vi "Front Panel Control Example.vi"() -> ()   [LabVIEW 2020]
uses:
  Controls/FP Control Functions.ctl
panel:
  in  "stop":bool
  # "While the VI is running, open the block diagram (Ctrl-E) and wait."
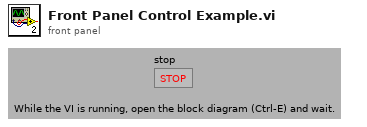
[diagram p1: front panel]
types:
  T1 = typedef "FP Control Functions.ctl" = enum16{"Open", "Close", "Bring To Front", "Center"}
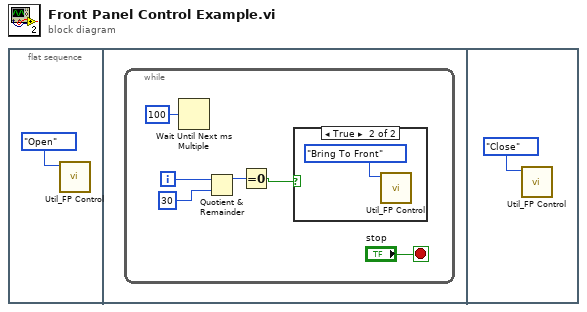
[diagram p0: block diagram]
diagram:
  n1 = flat-sequence {
    frame #0 {
      n2 = call "Util_FP Control.vi"("Function"=FP_Control_Functions."Open") -> ()  [unwired: 1 in, 10 out]
    }
    frame #1 {
      n3 = while {
        i -> [w5]
        stop <- "stop" stop-if-true
        n4 = Wait Until Next ms Multiple(millisecond multiple=u32 100) -> ()  [unwired: 1 out]
        n5 = Quotient & Remainder(x=w5, y=30) -> (x-y*floor(x/y)=w3:i32)  [unwired: 1 out]
        n6 = Equal To 0?(x=w3) -> (x = 0?=w2:bool)
        n7 = case shown="True" w2 {
          frame False {
          }
          frame True {
            n8 = call "Util_FP Control.vi"("Function"=FP_Control_Functions."Bring To Front") -> ()  [unwired: 1 in, 10 out]
          }
        }
      }
    }
    frame #2 {
      n9 = call "Util_FP Control.vi"("Function"=FP_Control_Functions."Close") -> ()  [unwired: 1 in, 10 out]
    }
  }
